vi "APC_9056_WarningIntegration.vi"(0 "NI9205":dbl[](array[numeric])=[-0.00361437722, 5.001652418760002, 9.99553711734999, 14.990208086199992, 19.993287157860003, 24.99203765954996, 29.986607142530012, 34.99718714015995, -0.001139086, -0.009304434079999986, -2.86875499999999e-05, 0.003279013959999996, -0.0027344005399999993, -0.0021136663599999996, -6.22128e-05, -0.006222946800000002] format="%0.2f", 1 "CURRENT SYSTEM STATE":i8, 2 "NI9208":dbl[](array[numeric])=[-0.0033997970000000004, 4.9987908475000005, 9.990422618, 14.998184486000001, 20.01738117, 25.004057022, 29.988959596500003, 34.99554141, -7.563000000000014e-05, 0.0006727460000000001, -0.0045439285, -0.007908694, -0.0070815059999999996, -0.00245116, 0.008481419, -0.011168849500000001] format="%0.5f", 3 "NI9214":dbl[](array[numeric])=[0.0010449026000000034, 4.999450598799999, 10.0006558688, 14.981061165000003] format="%0.2f", 4 "input cluster":T1, 5 "SYSTEM SIGNALS":dbl[](array[numeric])=[0.0, 0.0, 0.0, 0.0, 0.0, 0.0, 0.0, 0.0, 0.0, 0.0, 0.0, 0.0, 0.0, 0.0, 0.0, 0.0], 7 "LoadIni?":bool) -> (6 "STATE LIMITATION FROM WARNINGS":i8)   [LabVIEW 2020]
uses:
  controls/APC_WarningLimits.ctl
  controls/APC_PIDCluster.ctl
  <vilib>/Utility/xml.llb/Write to XML File(string).vi
  <vilib>/Utility/xml.llb/Read From XML File(string).vi
panel:
  in  "WarningLimits":T2={"Raster1_limits"=[[0.0, 10.0, 8.0, 12.0, 0.0, 0.0, 0.0, 0.0, 0.0, 0.0, 0.0, 0.0, 0.0, 0.0, 0.0, 0.0], [1.0, 8.0, 9.0, 13.0, 0.0, 0.0, 0.0, 0.0, 0.0, 0.0, 0.0, 0.0, 0.0, 0.0, 0.0, 0.0], [2.0, 7.0, 10.0, 14.0, 0.0, 0.0, 0.0, 0.0, 0.0, 0.0, 0.0, 0.0, 0.0, 0.0, 0.0, 0.0], [3.0, 6.0, 11.0, 15.0, 0.0, 0.0, 0.0, 0.0, 0.0, 0.0, 0.0, 0.0, 0.0, 0.0, 0.0, 150.0]], "Raster2_limits"=[[1.0, 0.0, 0.0, 0.0, 0.0, 0.0, 0.0, 0.0, 0.0, 0.0, 0.0, 0.0, 0.0, 0.0, 0.0, 0.0], [0.0, 0.0, 0.0, 0.0, 0.0, 0.0, 0.0, 0.0, 0.0, 0.0, 0.0, 0.0, 0.0, 0.0, 0.0, 0.0], [0.0, 0.0, 0.0, 0.0, 0.0, 0.0, 0.0, 0.0, 0.0, 0.0, 0.0, 0.0, 0.0, 0.0, 0.0, 0.0], [0.0, 0.0, 0.0, 0.0, 0.0, 0.0, 0.0, 0.0, 0.0, 0.0, 0.0, 0.0, 0.0, 0.0, 0.0, 0.0]], "Raster3_limits"=[[0.0, 10.0, 10.0, 0.0, 0.0, 0.0, 0.0, 0.0, 0.0, 0.0, 0.0, 0.0, 0.0, 0.0, 0.0, 0.0], [0.0, 9.0, 0.0, 0.0, 0.0, 0.0, 0.0, 0.0, 0.0, 0.0, 0.0, 0.0, 0.0, 0.0, 0.0, 0.0], [0.0, 7.0, 0.0, 0.0, 0.0, 0.0, 0.0, 0.0, 0.0, 0.0, 0.0, 0.0, 0.0, 0.0, 0.0, 0.0], [0.0, 5.5, 0.0, 0.0, 0.0, 0.0, 0.0, 0.0, 0.0, 0.0, 0.0, 0.0, 0.0, 0.0, 0.0, 0.0]], "Raster1_Sign"=[0.0, 0.0, 0.0, 0.0, 0.0, 0.0, 0.0, 0.0, 0.0, 0.0, 0.0, 0.0, 0.0, 0.0, 0.0, 0.0], "Raster2_Sign"=[0.0, 0.0, 0.0, 0.0, 0.0, 0.0, 0.0, 0.0, 0.0, 0.0, 0.0, 0.0, 0.0, 0.0, 0.0, 0.0], "Raster3_Sign"=[0.0, 0.0, 0.0, 0.0, 0.0, 0.0, 0.0, 0.0, 0.0, 0.0, 0.0, 0.0, 0.0, 0.0, 0.0, 0.0], "Raster4_Sign"=[0.0, 0.0, 0.0, 0.0, 0.0, 0.0, 0.0, 0.0, 0.0, 0.0, 0.0, 0.0, 0.0, 0.0, 0.0, 0.0], "Raster5_Sign"=[0.0, 0.0, 0.0, 0.0, 0.0, 0.0, 0.0, 0.0, 0.0, 0.0, 0.0, 0.0, 0.0, 0.0, 0.0, 0.0], "Raster5_limits"=[[0.0, 10.0, 10.0, 0.0, 0.0, 0.0, 0.0, 0.0, 0.0, 0.0, 0.0, 0.0, 0.0, 0.0, 0.0, 0.0], [0.0, 9.0, 0.0, 0.0, 0.0, 0.0, 0.0, 0.0, 0.0, 0.0, 0.0, 0.0, 0.0, 0.0, 0.0, 0.0], [0.0, 7.0, 0.0, 0.0, 0.0, 0.0, 0.0, 0.0, 0.0, 0.0, 0.0, 0.0, 0.0, 0.0, 0.0, 0.0], [0.0, 5.5, 0.0, 0.0, 0.0, 0.0, 0.0, 0.0, 0.0, 0.0, 0.0, 0.0, 0.0, 0.0, 0.0, 0.0]], "Raster4_limits"=[[0.0, 10.0, 10.0, 0.0, 0.0, 0.0, 0.0, 0.0, 0.0, 0.0, 0.0, 0.0, 0.0, 0.0, 0.0, 0.0], [0.0, 9.0, 0.0, 0.0, 0.0, 0.0, 0.0, 0.0, 0.0, 0.0, 0.0, 0.0, 0.0, 0.0, 0.0, 0.0], [0.0, 7.0, 0.0, 0.0, 0.0, 0.0, 0.0, 0.0, 0.0, 0.0, 0.0, 0.0, 0.0, 0.0, 0.0, 0.0], [0.0, 5.5, 0.0, 0.0, 0.0, 0.0, 0.0, 0.0, 0.0, 0.0, 0.0, 0.0, 0.0, 0.0, 0.0, 0.0]]}
  in  "load":bool
  out "MaxPress":u8
  out "Misfire":u8
  out "CyclicVar":u8
  out "Knock":u8
  out "LateComb":u8
  out "9049 not responding":bool
  out "9056 FPGA not responding":bool
  out "MergedCylinderErrors":u8[](array[numeric])
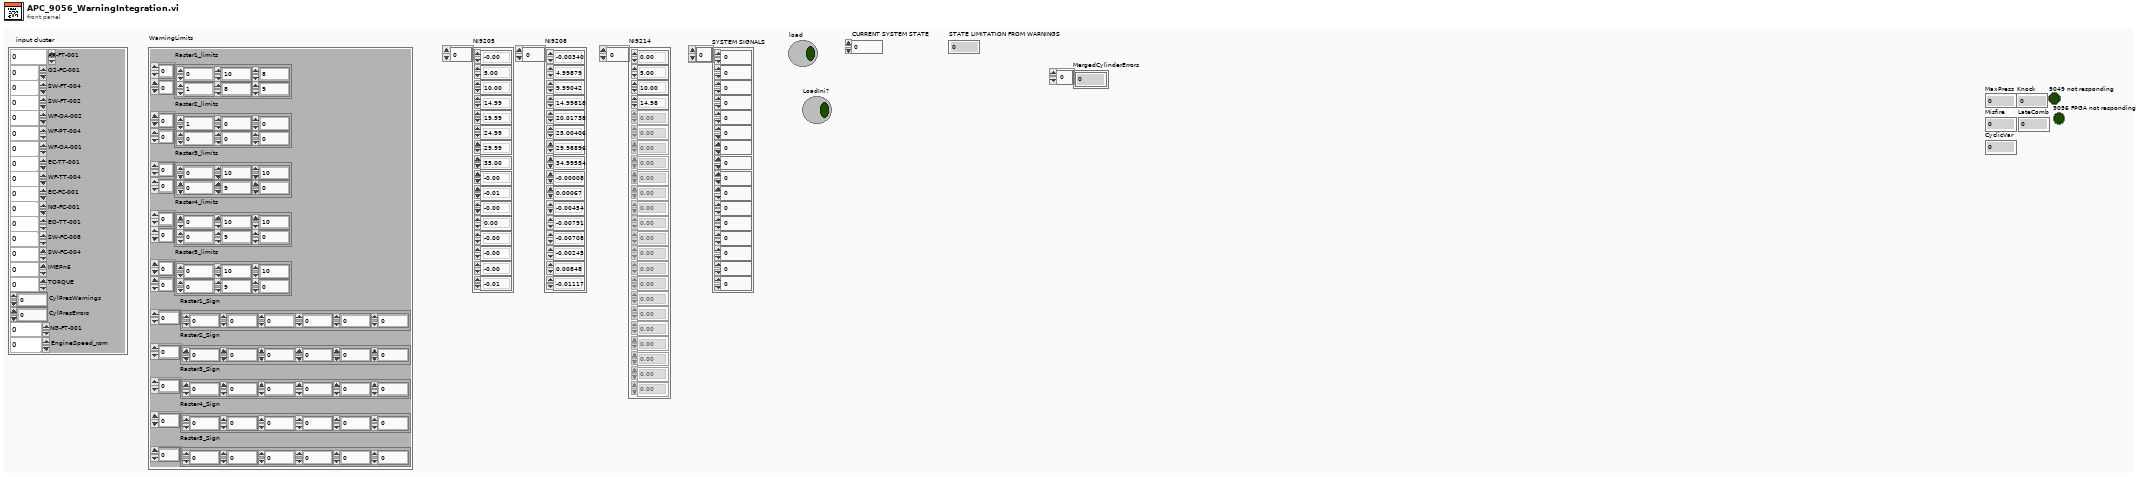
[diagram p1: front panel]
types:
  T1 = typedef "APC_PIDCluster.ctl" = cluster{"AR-FT-001":dbl, "O2-FC-001":dbl, "SW-FT-004":dbl, "SW-FT-002":dbl, "WF-OA-002":dbl, "WF-PT-004":dbl, "WF-OA-001":dbl, "EC-TT-001":dbl, "WF-TT-004":dbl, "EC-FC-001":dbl, "NG-FC-001":dbl, "EO-TT-001":dbl, "SW-FC-008":dbl, "SW-FC-004":dbl, "IMEPn6":dbl, "TORQUE":dbl, "CylPresWarnings":dbl, "CylPresErrors":dbl, "NG-FT-001":dbl, "EngineSpeed_rpm":dbl}
  T2 = typedef "APC_WarningLimits.ctl" = cluster{"Raster1_limits":dbl[][], "Raster2_limits":dbl[][], "Raster3_limits":dbl[][], "Raster1_Sign":dbl[], "Raster2_Sign":dbl[], "Raster3_Sign":dbl[], "Raster4_Sign":dbl[], "Raster5_Sign":dbl[], "Raster5_limits":dbl[][], "Raster4_limits":dbl[][]}
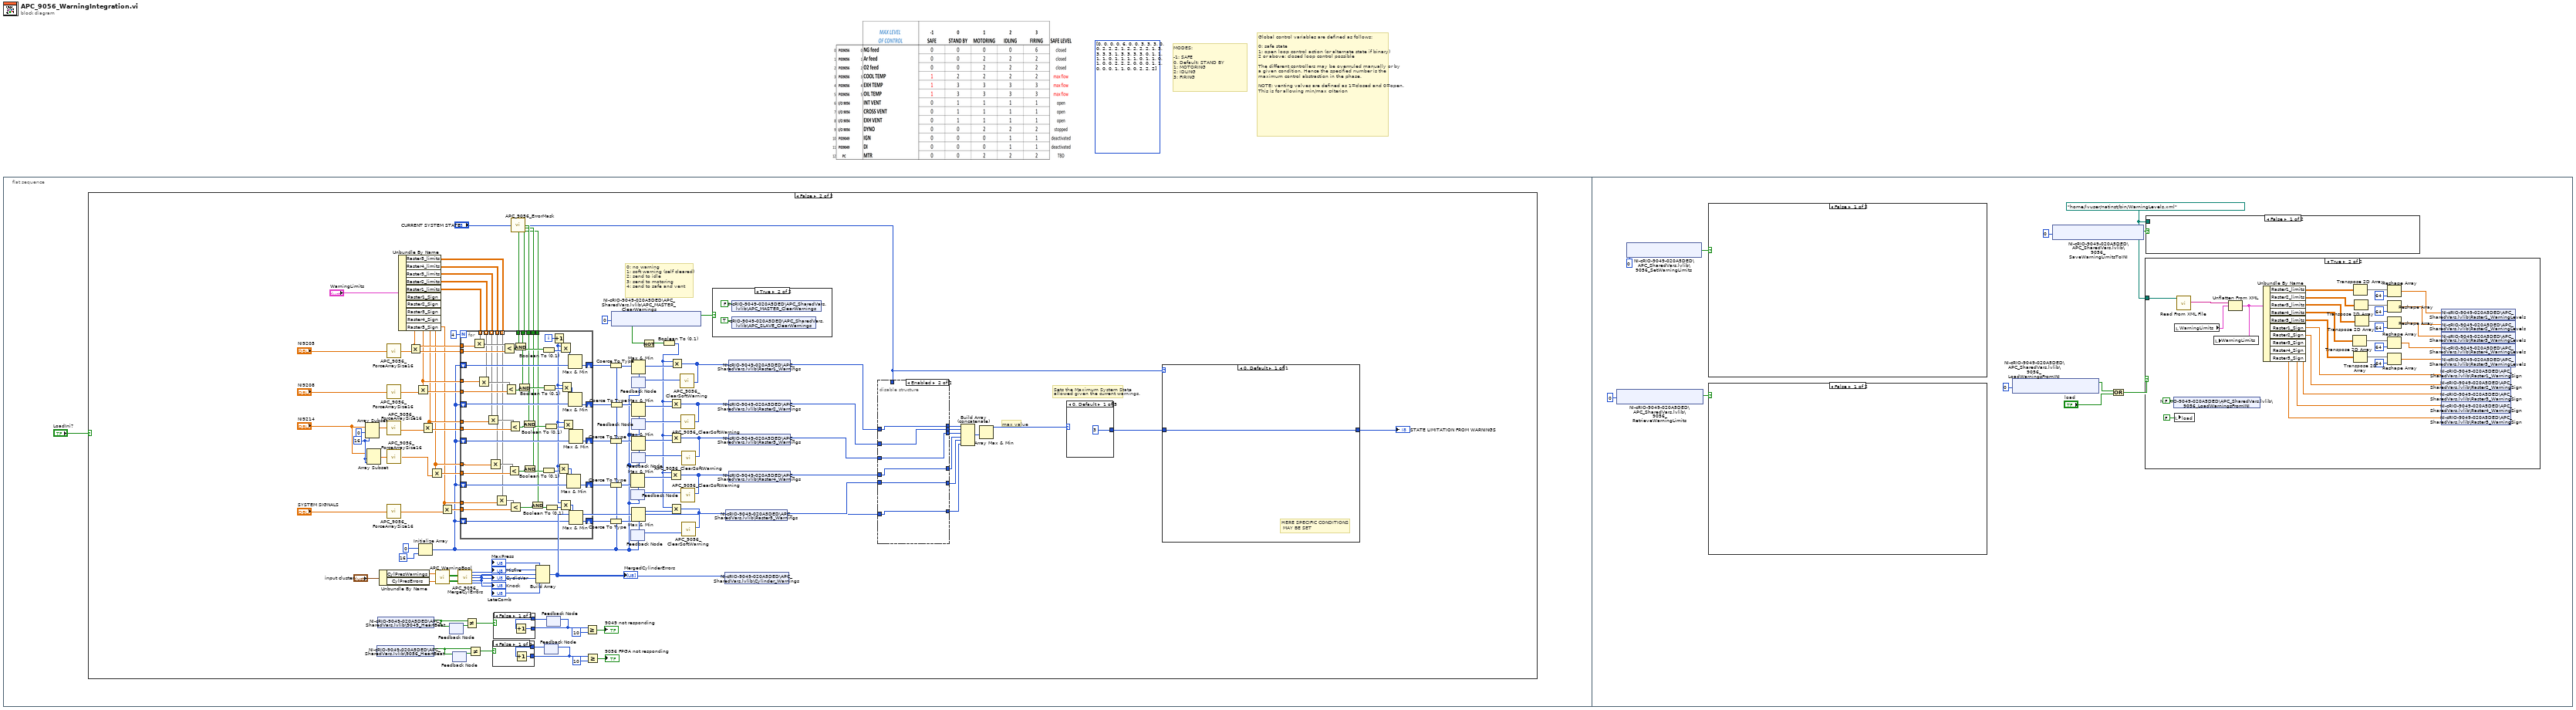
[diagram p0: block diagram]
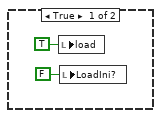
[diagram p2: hidden frame]
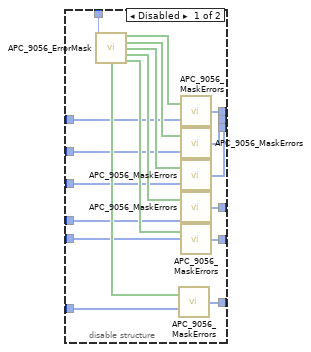
[diagram p3: hidden frame]
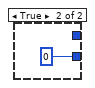
[diagram p4: hidden frame]
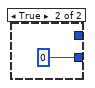
[diagram p5: hidden frame]
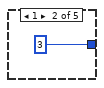
[diagram p7: hidden frame]
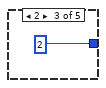
[diagram p8: hidden frame]
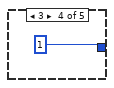
[diagram p9: hidden frame]
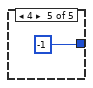
[diagram p10: hidden frame]
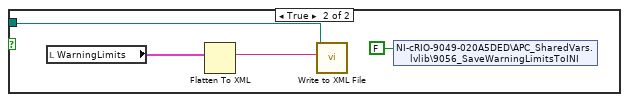
[diagram p12: hidden frame]
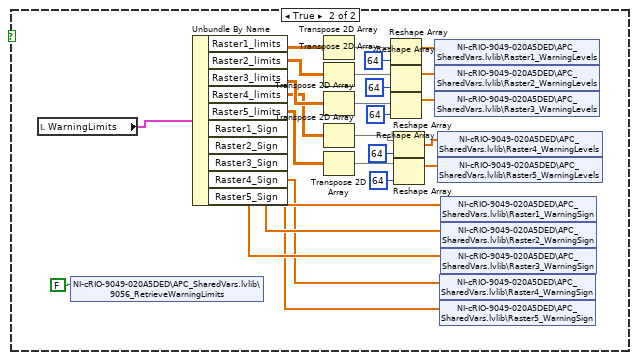
[diagram p13: hidden frame]
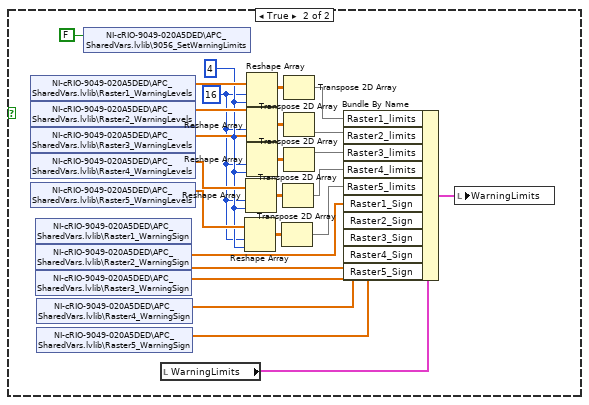
[diagram p14: hidden frame]
diagram:
  (unwired) i32[][] [[0, 0, 0, 0, 6], [0, 0, 3, 3, 3], [0, 0, 2, 2, 2], [1, 2, 2, 2, 2], [1, 3, 3, 3, 3], [1, 3, 3, 3, 3], [0, 1, 1, 1, 1], [0, 1, 1, 1, 1], [0, 1, 1, 0, 1], [0, 0, 2, 2, 2], [0, 0, 0, 1, 1], [0, 0, 0, 1, 1], [0, 0, 2, 2, 2]]
  # "Global control variables are defined as follows:\n\n0: safe state\n1: open loop control action (or alternate state if binary)\n2 or above: closed loop control possible\n\nThe different controllers may be overrruled manually or by a given condition. Hence the specified number is the maximum control abstraction in the phase.\n\nNOTE: venting valves are defined as 1=closed and 0=open. This is for allowing min/max criterion"
  # "MODES:\n\n-1: SAFE\n0, Default: STAND BY\n1: MOTORING\n2: IDLING\n3: FIRING"
  n1 = flat-sequence {
    frame #0 {
      n2 = case shown="False" "LoadIni?" {
        frame True {
          n3 = local write "load"(TRUE ("load")) -> ()
          n4 = local write "LoadIni?"(FALSE ("LoadIni?")) -> ()
        }
        frame False {
          w34 = 16 ("length")
          # "max value"
          # "Sets the Maximum System State allowed given the current warnings."
          # "0: no warning\n1: soft warning (self cleared)\n2: send to idle\n3: send to motoring\n4: send to safe and vent"
          n5 = Array Subset(array="NI9214", index=0, length=w34) -> (w5:dbl[])
          n6 = Array Subset(array="NI9214", index=w34, length=w34) -> (w7:dbl[])
          n7 = shared-variable "NI-cRIO-9049-020A5DED\\APC_SharedVars.lvlib\\9056_HeartBeat"() -> (w60:bool)  [unwired: 1 in, 1 out]
          n8 = shared-variable "NI-cRIO-9049-020A5DED\\APC_SharedVars.lvlib\\9049_HeartBeat"() -> (w63:bool)  [unwired: 1 in, 1 out]
          n9 = Unbundle By Name("input cluster") -> ("CylPresWarnings"=w19:dbl, "CylPresErrors"=w18:dbl)
          n10 = call "APC_9056_ForceArraySize16.vi"("ArrayIn"="NI9205") -> ("ArraOut"=w12:dbl[])
          n11 = call "APC_9056_ForceArraySize16.vi"("ArrayIn"="NI9208") -> ("ArraOut"=w10:dbl[])
          n12 = call "APC_9056_ForceArraySize16.vi"("ArrayIn"=w5) -> ("ArraOut"=w4:dbl[])
          n13 = call "APC_9056_ForceArraySize16.vi"("ArrayIn"=w7) -> ("ArraOut"=w6:dbl[])
          n14 = call "APC_9056_ForceArraySize16.vi"("ArrayIn"="SYSTEM SIGNALS") -> ("ArraOut"=w8:dbl[])
          n15 = Unbundle By Name("WarningLimits") -> ("Raster5_limits"=w48:dbl[][], "Raster4_limits"=w49:dbl[][], "Raster3_limits"=w98:dbl[][], "Raster2_limits"=w97:dbl[][], "Raster1_limits"=w96:dbl[][], "Raster1_Sign"=w78:dbl[], "Raster2_Sign"=w77:dbl[], "Raster3_Sign"=w76:dbl[], "Raster4_Sign"=w46:dbl[], "Raster5_Sign"=w43:dbl[])
          n16 = Multiply(x=w78, y=w12) -> (x*y=w81:dbl[])
          n17 = Multiply(x=w77, y=w10) -> (x*y=w80:dbl[])
          n18 = Initialize Array(u8 0 ("element"), 16 ("dimension size")) -> (w14:u8[])
          n19 = Multiply(x=w76, y=w4) -> (x*y=w79:dbl[])
          n20 = Multiply(x=w46, y=w6) -> (x*y=w47:dbl[])
          n21 = call "APC_WarningBool.vi"("CylPresErrors"=w18, "CylPresWarnings"=w19) -> ("Error"=w15:bool[][], "Warning"=w16:bool[][])
          n22 = Multiply(x=w43, y=w8) -> (x*y=w44:dbl[])
          n23 = feedback #1() -> (w62:bool)  [unwired: 1 in]
          n24 = feedback-in #1(w63) -> ()
          n25 = feedback #2() -> (w61:bool)  [unwired: 1 in]
          n26 = feedback-in #2(w60) -> ()
          n27 = call "APC_9056_MergeCylErrors.vi"("CylPressWarning"=w16, "CylPressError"=w15) -> ("MaxPress"=w68:u8, "Misfire (1 to 3)"=w67:u8, "CyclicVar"=w66:u8, "Knock"=w65:u8, "LateComb"=w64:u8)  [unwired: 9 in]
          "MaxPress" <- w68
          "Misfire" <- w67
          "CyclicVar" <- w66
          "Knock" <- w65
          "LateComb" <- w64
          n28 = Not Equal?(x=w63, y=w62) -> (x != y?=w59:bool)
          n29 = Not Equal?(x=w60, y=w61) -> (x != y?=w58:bool)
          n30 = call "APC_9056_ErrorMask.vi"("SYSTEM STATE"="CURRENT SYSTEM STATE") -> ("raster1mask"=w75:bool[], "raster2mask"=w74:bool[], "raster3mask"=w73:bool[], "raster4mask"=w45:bool[], "raster5mask"=w42:bool[])  [unwired: 9 in, 1 out]
          n31 = for {
            N: 4 -> [_]
            tunnel: w96 -> [w183] mode=indexing
            tunnel: w81 -> [w200]
            shift-right: [w194] -> w87
            shift-left: w14 -> [w201]
            shift-right: [w195] -> w84
            shift-left: w14 -> [w193]
            tunnel: w80 -> [w192]
            shift-right: [w189] -> w82
            shift-left: w14 -> [w188]
            tunnel: w79 -> [w187]
            tunnel: w97 -> [w180] mode=indexing
            tunnel: w98 -> [w178] mode=indexing
            tunnel: w78 -> [w184]
            tunnel: w77 -> [w181]
            tunnel: w76 -> [w177]
            tunnel: w75 -> [w170]
            tunnel: w74 -> [w169]
            tunnel: w73 -> [w168]
            tunnel: w49 -> [w148] mode=indexing
            tunnel: w48 -> [w147] mode=indexing
            shift-right: [w162] -> w33
            shift-left: w14 -> [w159]
            tunnel: w47 -> [w161]
            tunnel: w46 -> [w160]
            tunnel: w45 -> [w158]
            shift-right: [w152] -> w31
            shift-left: w14 -> [w151]
            tunnel: w44 -> [w150]
            tunnel: w43 -> [w149]
            tunnel: w42 -> [w146]
            i -> [w186]
            n32 = Multiply(x=w183, y=w184) -> (x*y=w185:dbl[])
            n33 = Multiply(x=w180, y=w181) -> (x*y=w182:dbl[])
            n34 = Multiply(x=w178, y=w177) -> (x*y=w179:dbl[])
            n35 = Multiply(x=w148, y=w160) -> (x*y=w165:dbl[])
            n36 = Multiply(x=w147, y=w149) -> (x*y=w155:dbl[])
            n37 = Less?(x=w185, y=w200) -> (x < y?=w176:bool[])
            n38 = Less?(x=w182, y=w192) -> (x < y?=w174:bool[])
            n39 = Less?(x=w165, y=w161) -> (x < y?=w164:bool[])
            n40 = Less?(x=w179, y=w187) -> (x < y?=w172:bool[])
            n41 = Less?(x=w155, y=w150) -> (x < y?=w154:bool[])
            n42 = And(x=w170, y=w176) -> (x .and. y?=w175:bool[])
            n43 = And(x=w169, y=w174) -> (x .and. y?=w173:bool[])
            n44 = And(x=w168, y=w172) -> (x .and. y?=w171:bool[])
            n45 = And(x=w158, y=w164) -> (x .and. y?=w163:bool[])
            n46 = And(x=w146, y=w154) -> (x .and. y?=w153:bool[])
            n47 = Boolean To (0,1)(Boolean=w175) -> (0, 1=w199:i16[])
            n48 = Boolean To (0,1)(Boolean=w163) -> (0, 1=w167:i16[])
            n49 = Boolean To (0,1)(Boolean=w173) -> (0, 1=w197:i16[])
            n50 = Boolean To (0,1)(Boolean=w171) -> (0, 1=w191:i16[])
            n51 = Boolean To (0,1)(Boolean=w153) -> (0, 1=w157:i16[])
            n52 = Increment(x=w186) -> (x+1=w145:i32)
            n53 = Multiply(x=w145, y=w167) -> (x*y=w166:i32[])
            n54 = Multiply(x=w145, y=w199) -> (x*y=w198:i32[])
            n55 = Multiply(x=w145, y=w157) -> (x*y=w156:i32[])
            n56 = Multiply(x=w145, y=w197) -> (x*y=w196:i32[])
            n57 = Multiply(x=w145, y=w191) -> (x*y=w190:i32[])
            n58 = Max & Min(x=w166, y=w159) -> (min(x,y)=w162:i32[])  [unwired: 1 out]
            n59 = Max & Min(x=w198, y=w201) -> (max(x,y)=w194:i32[])  [unwired: 1 out]
            n60 = Max & Min(x=w196, y=w193) -> (max(x,y)=w195:i32[])  [unwired: 1 out]
            n61 = Max & Min(x=w156, y=w151) -> (min(x,y)=w152:i32[])  [unwired: 1 out]
            n62 = Max & Min(x=w190, y=w188) -> (max(x,y)=w189:i32[])  [unwired: 1 out]
          }
          n63 = Build Array(w68, w67, w66, w65, w64) -> (w22:u8[])
          "MergedCylinderErrors" <- w22
          n64 = feedback #3() -> (w56:i32)  [unwired: 1 in]
          n65 = case shown="False" w58 {
            tunnel: [w138 0] -> w52
            tunnel: w56 -> [w137 _]
            frame False {
              n66 = Increment(x=w137) -> (x+1=w138:i32)
            }
            frame True {
            }
          }
          n67 = feedback-in #3(w52) -> ()
          n68 = feedback #4() -> (w57:i32)  [unwired: 1 in]
          n69 = case shown="False" w59 {
            tunnel: [w141 0] -> w55
            tunnel: w57 -> [w140 _]
            frame False {
              n70 = Increment(x=w140) -> (x+1=w141:i32)
            }
            frame True {
            }
          }
          n71 = feedback-in #4(w55) -> ()
          n72 = Greater Or Equal?(x=w55, y=10) -> (x >= y?=→"9049 not responding":bool)
          n73 = Greater Or Equal?(x=w52, y=10) -> (x >= y?=→"9056 FPGA not responding":bool)
          n74 = Coerce To Type(0:w87, 1:w14) -> (2:w86:u8[])
          n75 = Coerce To Type(0:w82, 1:w14) -> (2:w85:u8[])
          n76 = Coerce To Type(0:w33, 1:w14) -> (2:w32:u8[])
          n77 = Coerce To Type(0:w31, 1:w14) -> (2:w30:u8[])
          n78 = Coerce To Type(0:w84, 1:w14) -> (2:w83:u8[])
          n79 = shared-variable "NI-cRIO-9049-020A5DED\\APC_SharedVars.lvlib\\APC_MASTER_ClearWarnings"(0 ("ms timeout (0)")) -> (w89:bool)  [unwired: 1 in, 2 out]
          n80 = feedback #5(w14) -> (w41:u8[])
          n81 = Max & Min(x=w32, y=w41) -> (max(x,y)=w40:u8[])  [unwired: 1 out]
          n82 = feedback #6(w14) -> (w36:u8[])
          n83 = feedback #7(w14) -> (w95:u8[])
          n84 = Max & Min(x=w86, y=w95) -> (max(x,y)=w92:u8[])  [unwired: 1 out]
          n85 = feedback #8(w14) -> (w94:u8[])
          n86 = Max & Min(x=w83, y=w94) -> (max(x,y)=w91:u8[])  [unwired: 1 out]
          n87 = feedback #9(w14) -> (w93:u8[])
          n88 = Max & Min(x=w85, y=w93) -> (max(x,y)=w90:u8[])  [unwired: 1 out]
          n89 = Max & Min(x=w30, y=w36) -> (max(x,y)=w38:u8[])  [unwired: 1 out]
          n90 = Not(x=w89) -> (.not. x?=w69:bool)
          n91 = Boolean To (0,1)(Boolean=w69) -> (0, 1=w29:i16)
          n92 = Multiply(x=w29, y=w40) -> (x*y=w24:i16[])
          n93 = Multiply(x=w29, y=w91) -> (x*y=w26:i16[])
          n94 = Multiply(x=w29, y=w90) -> (x*y=w25:i16[])
          n95 = Multiply(x=w29, y=w38) -> (x*y=w23:i16[])
          n96 = Multiply(x=w29, y=w92) -> (x*y=w27:i16[])
          n97 = call "APC_9056_ClearSoftWarning.vi"("WarningIn"=w27) -> ("WarningOut"=w72:u8[])
          n98 = feedback-in #7(w72) -> ()
          n99 = call "APC_9056_ClearSoftWarning.vi"("WarningIn"=w26) -> ("WarningOut"=w71:u8[])
          n100 = feedback-in #8(w71) -> ()
          n101 = call "APC_9056_ClearSoftWarning.vi"("WarningIn"=w24) -> ("WarningOut"=w39:u8[])
          n102 = feedback-in #5(w39) -> ()
          n103 = call "APC_9056_ClearSoftWarning.vi"("WarningIn"=w25) -> ("WarningOut"=w70:u8[])
          n104 = feedback-in #9(w70) -> ()
          n105 = call "APC_9056_ClearSoftWarning.vi"("WarningIn"=w23) -> ("WarningOut"=w37:u8[])
          n106 = feedback-in #6(w37) -> ()
          n107 = case shown="True" w89 {
            frame False {
            }
            frame True {
              n108 = shared-variable "NI-cRIO-9049-020A5DED\\APC_SharedVars.lvlib\\APC_MASTER_ClearWarnings"(FALSE ("Clear9056warnings")) -> ()  [unwired: 1 in, 1 out]
              n109 = shared-variable "NI-cRIO-9049-020A5DED\\APC_SharedVars.lvlib\\APC_SLAVE_ClearWarnings"(TRUE ("Clear9056warnings")) -> ()  [unwired: 1 in, 1 out]
            }
          }
          n110 = shared-variable "NI-cRIO-9049-020A5DED\\APC_SharedVars.lvlib\\Cylinder_Warnings"(w22) -> ()  [unwired: 1 in, 1 out]
          n111 = shared-variable "NI-cRIO-9049-020A5DED\\APC_SharedVars.lvlib\\Raster5_Warnings"(w23) -> ()  [unwired: 1 in, 1 out]
          n112 = shared-variable "NI-cRIO-9049-020A5DED\\APC_SharedVars.lvlib\\Raster1_Warnings"(w27) -> ()  [unwired: 1 in, 1 out]
          n113 = shared-variable "NI-cRIO-9049-020A5DED\\APC_SharedVars.lvlib\\Raster2_Warnings"(w26) -> ()  [unwired: 1 in, 1 out]
          n114 = shared-variable "NI-cRIO-9049-020A5DED\\APC_SharedVars.lvlib\\Raster3_Warnings"(w25) -> ()  [unwired: 1 in, 1 out]
          n115 = shared-variable "NI-cRIO-9049-020A5DED\\APC_SharedVars.lvlib\\Raster4_Warnings"(w24) -> ()  [unwired: 1 in, 1 out]
          n116 = disable-structure shown="Enabled" {
            disable-tunnel: [w125 w136] -> w111
            disable-tunnel: [w124 w135] -> w110
            disable-tunnel: [w123 w134] -> w109
            disable-tunnel: [w122 w133] -> w108
            disable-tunnel: [w121 w132] -> w107
            disable-tunnel: [w119 w131] -> w102
            disable-tunnel: w27 -> [w118 w136]
            disable-tunnel: w26 -> [w117 w135]
            disable-tunnel: w25 -> [w116 w134]
            disable-tunnel: w24 -> [w115 w133]
            disable-tunnel: w23 -> [w114 w132]
            disable-tunnel: w22 -> [w113 w131]
            disable-tunnel: "CURRENT SYSTEM STATE" -> [w112 _]
            frame Disabled {
              n117 = call "APC_9056_ErrorMask.vi"("SYSTEM STATE"=w112) -> ("raster1mask"=w130:bool[], "raster2mask"=w129:bool[], "raster3mask"=w128:bool[], "raster4mask"=w127:bool[], "CylinderMask"=w120:bool[], "raster5mask"=w126:bool[])  [unwired: 9 in]
              n118 = call "APC_9056_MaskErrors.vi"("UnMaskedWarning"=w113, "rastermask"=w120) -> ("MaskedWarning"=w119:u8[])
              n119 = call "APC_9056_MaskErrors.vi"("UnMaskedWarning"=w118, "rastermask"=w130) -> ("MaskedWarning"=w125:u8[])
              n120 = call "APC_9056_MaskErrors.vi"("UnMaskedWarning"=w117, "rastermask"=w129) -> ("MaskedWarning"=w124:u8[])
              n121 = call "APC_9056_MaskErrors.vi"("UnMaskedWarning"=w116, "rastermask"=w128) -> ("MaskedWarning"=w123:u8[])
              n122 = call "APC_9056_MaskErrors.vi"("UnMaskedWarning"=w115, "rastermask"=w127) -> ("MaskedWarning"=w122:u8[])
              n123 = call "APC_9056_MaskErrors.vi"("UnMaskedWarning"=w114, "rastermask"=w126) -> ("MaskedWarning"=w121:u8[])
            }
            frame Enabled {
            }
          }
          n124 = Build Array (concatenate)(w111, w110, w109, w108, w107, w102) -> (w106:i16[])
          n125 = Array Max & Min(array=w106) -> (max value=w105:i16)  [unwired: 3 out]
          n126 = case shown="0, Default" w105 {
            tunnel: [i8 3 i8 3 i8 2 i8 1 i8 -1] -> w104
            frame 0, Default {
            }
            frame 1 {
            }
            frame 2 {
            }
            frame 3 {
            }
            frame 4 {
            }
          }
          n127 = case shown="0, Default" "CURRENT SYSTEM STATE" {
            tunnel: w104 -> [w207]
            tunnel: [w207] -> w103
            frame 0, Default {
              # "HERE SPECIFIC CONDITIONS\n MAY BE SET"
            }
          }
          "STATE LIMITATION FROM WARNINGS" <- w103
        }
      }
    }
    frame #1 {
      w212 = path "/home/lvuser/natinst/bin/WarningLevels.xml" ("XML File Path")
      n128 = shared-variable "NI-cRIO-9049-020A5DED\\APC_SharedVars.lvlib\\9056_RetrieveWarningLimits"(0 ("ms timeout (0)")) -> (w216:bool)  [unwired: 1 in, 2 out]
      n129 = shared-variable "NI-cRIO-9049-020A5DED\\APC_SharedVars.lvlib\\9056_SetWarningLimits"(0 ("ms timeout (0)")) -> (w217:bool)  [unwired: 1 in, 2 out]
      n130 = case shown="False" w217 {
        frame False {
        }
        frame True {
          w286 = 4 ("dimension size")
          w285 = 16 ("dimension size")
          n131 = shared-variable "NI-cRIO-9049-020A5DED\\APC_SharedVars.lvlib\\Raster1_WarningLevels"() -> (w304:dbl[])  [unwired: 1 in, 1 out]
          n132 = shared-variable "NI-cRIO-9049-020A5DED\\APC_SharedVars.lvlib\\Raster2_WarningLevels"() -> (w303:dbl[])  [unwired: 1 in, 1 out]
          n133 = shared-variable "NI-cRIO-9049-020A5DED\\APC_SharedVars.lvlib\\Raster3_WarningLevels"() -> (w302:dbl[])  [unwired: 1 in, 1 out]
          n134 = shared-variable "NI-cRIO-9049-020A5DED\\APC_SharedVars.lvlib\\Raster4_WarningLevels"() -> (w288:dbl[])  [unwired: 1 in, 1 out]
          n135 = shared-variable "NI-cRIO-9049-020A5DED\\APC_SharedVars.lvlib\\Raster5_WarningLevels"() -> (w287:dbl[])  [unwired: 1 in, 1 out]
          n136 = shared-variable "NI-cRIO-9049-020A5DED\\APC_SharedVars.lvlib\\Raster1_WarningSign"() -> (w293:dbl[])  [unwired: 1 in, 1 out]
          n137 = shared-variable "NI-cRIO-9049-020A5DED\\APC_SharedVars.lvlib\\Raster2_WarningSign"() -> (w294:dbl[])  [unwired: 1 in, 1 out]
          n138 = shared-variable "NI-cRIO-9049-020A5DED\\APC_SharedVars.lvlib\\Raster3_WarningSign"() -> (w295:dbl[])  [unwired: 1 in, 1 out]
          n139 = shared-variable "NI-cRIO-9049-020A5DED\\APC_SharedVars.lvlib\\Raster4_WarningSign"() -> (w292:dbl[])  [unwired: 1 in, 1 out]
          n140 = shared-variable "NI-cRIO-9049-020A5DED\\APC_SharedVars.lvlib\\Raster5_WarningSign"() -> (w291:dbl[])  [unwired: 1 in, 1 out]
          n141 = shared-variable "NI-cRIO-9049-020A5DED\\APC_SharedVars.lvlib\\9056_SetWarningLimits"(FALSE ("SetWarningLimits")) -> ()  [unwired: 1 in, 1 out]
          n142 = local read "WarningLimits"() -> (w282:T2)
          n143 = Reshape Array(w287, w285, w286) -> (w289:dbl[][])
          n144 = Reshape Array(w288, w285, w286) -> (w290:dbl[][])
          n145 = Reshape Array(w304, w285, w286) -> (w296:dbl[][])
          n146 = Reshape Array(w303, w285, w286) -> (w299:dbl[][])
          n147 = Reshape Array(w302, w285, w286) -> (w301:dbl[][])
          n148 = Transpose 2D Array(2D array=w289) -> (transposed array=w283:dbl[][])
          n149 = Transpose 2D Array(2D array=w290) -> (transposed array=w284:dbl[][])
          n150 = Transpose 2D Array(2D array=w296) -> (transposed array=w297:dbl[][])
          n151 = Transpose 2D Array(2D array=w299) -> (transposed array=w298:dbl[][])
          n152 = Transpose 2D Array(2D array=w301) -> (transposed array=w300:dbl[][])
          n153 = Bundle By Name(cluster=w282, "Raster1_limits"=w297, "Raster2_limits"=w298, "Raster3_limits"=w300, "Raster4_limits"=w284, "Raster5_limits"=w283, "Raster1_Sign"=w293, "Raster2_Sign"=w294, "Raster3_Sign"=w295, "Raster4_Sign"=w292, "Raster5_Sign"=w291) -> (w281:T2)
          n154 = local write "WarningLimits"(w281) -> ()
        }
      }
      n155 = case shown="False" w216 {
        frame False {
        }
        frame True {
          n156 = local read "WarningLimits"() -> (w254:T2)
          n157 = shared-variable "NI-cRIO-9049-020A5DED\\APC_SharedVars.lvlib\\9056_RetrieveWarningLimits"(FALSE ("RetrieveWarningLimits")) -> ()  [unwired: 1 in, 1 out]
          n158 = Unbundle By Name(w254) -> ("Raster1_limits"=w269:dbl[][], "Raster2_limits"=w271:dbl[][], "Raster3_limits"=w273:dbl[][], "Raster4_limits"=w258:dbl[][], "Raster5_limits"=w256:dbl[][], "Raster1_Sign"=w267:dbl[], "Raster2_Sign"=w266:dbl[], "Raster3_Sign"=w265:dbl[], "Raster4_Sign"=w264:dbl[], "Raster5_Sign"=w263:dbl[])
          n159 = Transpose 2D Array(2D array=w269) -> (transposed array=w268:dbl[][])
          n160 = Transpose 2D Array(2D array=w271) -> (transposed array=w270:dbl[][])
          n161 = Transpose 2D Array(2D array=w273) -> (transposed array=w272:dbl[][])
          n162 = Transpose 2D Array(2D array=w258) -> (transposed array=w257:dbl[][])
          n163 = Transpose 2D Array(2D array=w256) -> (transposed array=w255:dbl[][])
          n164 = Reshape Array(w268, 64 ("dimension size")) -> (w278:dbl[])
          n165 = Reshape Array(w270, 64 ("dimension size")) -> (w276:dbl[])
          n166 = Reshape Array(w272, 64 ("dimension size")) -> (w274:dbl[])
          n167 = Reshape Array(w257, 64 ("dimension size")) -> (w259:dbl[])
          n168 = Reshape Array(w255, 64 ("dimension size")) -> (w260:dbl[])
          n169 = shared-variable "NI-cRIO-9049-020A5DED\\APC_SharedVars.lvlib\\Raster1_WarningLevels"(w278) -> ()  [unwired: 1 in, 1 out]
          n170 = shared-variable "NI-cRIO-9049-020A5DED\\APC_SharedVars.lvlib\\Raster2_WarningLevels"(w276) -> ()  [unwired: 1 in, 1 out]
          n171 = shared-variable "NI-cRIO-9049-020A5DED\\APC_SharedVars.lvlib\\Raster3_WarningLevels"(w274) -> ()  [unwired: 1 in, 1 out]
          n172 = shared-variable "NI-cRIO-9049-020A5DED\\APC_SharedVars.lvlib\\Raster4_WarningLevels"(w259) -> ()  [unwired: 1 in, 1 out]
          n173 = shared-variable "NI-cRIO-9049-020A5DED\\APC_SharedVars.lvlib\\Raster5_WarningLevels"(w260) -> ()  [unwired: 1 in, 1 out]
          n174 = shared-variable "NI-cRIO-9049-020A5DED\\APC_SharedVars.lvlib\\Raster4_WarningSign"(w264) -> ()  [unwired: 1 in, 1 out]
          n175 = shared-variable "NI-cRIO-9049-020A5DED\\APC_SharedVars.lvlib\\Raster5_WarningSign"(w263) -> ()  [unwired: 1 in, 1 out]
          n176 = shared-variable "NI-cRIO-9049-020A5DED\\APC_SharedVars.lvlib\\Raster1_WarningSign"(w267) -> ()  [unwired: 1 in, 1 out]
          n177 = shared-variable "NI-cRIO-9049-020A5DED\\APC_SharedVars.lvlib\\Raster2_WarningSign"(w266) -> ()  [unwired: 1 in, 1 out]
          n178 = shared-variable "NI-cRIO-9049-020A5DED\\APC_SharedVars.lvlib\\Raster3_WarningSign"(w265) -> ()  [unwired: 1 in, 1 out]
        }
      }
      n179 = shared-variable "NI-cRIO-9049-020A5DED\\APC_SharedVars.lvlib\\9056_LoadWarningsFromINI"(0 ("ms timeout (0)")) -> (w209:bool)  [unwired: 1 in, 2 out]
      n180 = shared-variable "NI-cRIO-9049-020A5DED\\APC_SharedVars.lvlib\\9056_SaveWarningLimitsToINI"(0 ("ms timeout (0)")) -> (w214:bool)  [unwired: 1 in, 2 out]
      n181 = Or(x=w209, y="load") -> (x .or. y?=w210:bool)
      n182 = case shown="True" w210 {
        tunnel: w212 -> [_ w248]
        frame False {
        }
        frame True {
          n183 = shared-variable "NI-cRIO-9049-020A5DED\\APC_SharedVars.lvlib\\9056_LoadWarningsFromINI"(FALSE ("SetWarningLimits")) -> ()  [unwired: 1 in, 1 out]
          n184 = local write "load"(FALSE ("load")) -> ()
          n185 = local read "WarningLimits"() -> (w220:T2)
          n186 = call-poly <vilib>:"Read From XML File.vi"("XML File Path"=w248) -> ("XML Elements"=w249:string)  [unwired: 8 in, 2 out]
          n187 = Unflatten From XML(xml string=w249, type=w220) -> (value=w219:T2)  [unwired: 1 in, 1 out]
          n188 = local write "WarningLimits"(w219) -> ()
          n189 = Unbundle By Name(w219) -> ("Raster1_limits"=w241:dbl[][], "Raster2_limits"=w239:dbl[][], "Raster3_limits"=w237:dbl[][], "Raster4_limits"=w224:dbl[][], "Raster5_limits"=w223:dbl[][], "Raster1_Sign"=w235:dbl[], "Raster2_Sign"=w234:dbl[], "Raster3_Sign"=w233:dbl[], "Raster4_Sign"=w232:dbl[], "Raster5_Sign"=w231:dbl[])
          n190 = Transpose 2D Array(2D array=w224) -> (transposed array=w226:dbl[][])
          n191 = Transpose 2D Array(2D array=w223) -> (transposed array=w225:dbl[][])
          n192 = Transpose 2D Array(2D array=w241) -> (transposed array=w240:dbl[][])
          n193 = Transpose 2D Array(2D array=w239) -> (transposed array=w238:dbl[][])
          n194 = Transpose 2D Array(2D array=w237) -> (transposed array=w236:dbl[][])
          n195 = Reshape Array(w240, 64 ("dimension size")) -> (w246:dbl[])
          n196 = Reshape Array(w238, 64 ("dimension size")) -> (w244:dbl[])
          n197 = Reshape Array(w236, 64 ("dimension size")) -> (w242:dbl[])
          n198 = Reshape Array(w226, 64 ("dimension size")) -> (w229:dbl[])
          n199 = Reshape Array(w225, 64 ("dimension size")) -> (w227:dbl[])
          n200 = shared-variable "NI-cRIO-9049-020A5DED\\APC_SharedVars.lvlib\\Raster1_WarningLevels"(w246) -> ()  [unwired: 1 in, 1 out]
          n201 = shared-variable "NI-cRIO-9049-020A5DED\\APC_SharedVars.lvlib\\Raster2_WarningLevels"(w244) -> ()  [unwired: 1 in, 1 out]
          n202 = shared-variable "NI-cRIO-9049-020A5DED\\APC_SharedVars.lvlib\\Raster3_WarningLevels"(w242) -> ()  [unwired: 1 in, 1 out]
          n203 = shared-variable "NI-cRIO-9049-020A5DED\\APC_SharedVars.lvlib\\Raster4_WarningLevels"(w229) -> ()  [unwired: 1 in, 1 out]
          n204 = shared-variable "NI-cRIO-9049-020A5DED\\APC_SharedVars.lvlib\\Raster5_WarningLevels"(w227) -> ()  [unwired: 1 in, 1 out]
          n205 = shared-variable "NI-cRIO-9049-020A5DED\\APC_SharedVars.lvlib\\Raster1_WarningSign"(w235) -> ()  [unwired: 1 in, 1 out]
          n206 = shared-variable "NI-cRIO-9049-020A5DED\\APC_SharedVars.lvlib\\Raster2_WarningSign"(w234) -> ()  [unwired: 1 in, 1 out]
          n207 = shared-variable "NI-cRIO-9049-020A5DED\\APC_SharedVars.lvlib\\Raster3_WarningSign"(w233) -> ()  [unwired: 1 in, 1 out]
          n208 = shared-variable "NI-cRIO-9049-020A5DED\\APC_SharedVars.lvlib\\Raster4_WarningSign"(w232) -> ()  [unwired: 1 in, 1 out]
          n209 = shared-variable "NI-cRIO-9049-020A5DED\\APC_SharedVars.lvlib\\Raster5_WarningSign"(w231) -> ()  [unwired: 1 in, 1 out]
        }
      }
      n210 = case shown="False" w214 {
        tunnel: w212 -> [_ w251]
        frame False {
        }
        frame True {
          n211 = local read "WarningLimits"() -> (w250:T2)
          n212 = Flatten To XML(6:w250) -> (2:w252:string)
          n213 = call-poly <vilib>:"Write to XML File.vi"("XML Input"=w252, "XML File Path"=w251) -> ()  [unwired: 7 in, 3 out]
          n214 = shared-variable "NI-cRIO-9049-020A5DED\\APC_SharedVars.lvlib\\9056_SaveWarningLimitsToINI"(FALSE ("SetWarningLimits")) -> ()  [unwired: 1 in, 1 out]
        }
      }
    }
  }
